vi "daub4_DWT.vi"(10 "RMS":dbl[](array[numeric])) -> (2 "Wavelet Coeff":dbl[](array[numeric]))   [LabVIEW 2014]
uses:
  <vilib>/imath/engines/lvmath2/RunTimeEngine/Managers/WorkSpace/UID Generator.vi
  <vilib>/imath/engines/lvmath2/RunTimeEngine/RunTimeType/NIMS_RunTimeType_From StrictType (excl LVString).vi
  <instcachedir>/0/NIMS_RunTimeType_From StrictType (excl LVString)_15A5391EEA9C4AACB9955AC755B83D29.lvgen/NIMS_RunTimeType_From StrictType (excl LVString)_15A5391EEA9C4AACB9955AC755B83D29_000.vi
  <vilib>/imath/engines/lvmath2/RunTimeEngine/LocalVariableDefStatement/MC_LocalVariableDefStatement_Display.vi
  <vilib>/imath/engines/lvmath2/RunTimeEngine/BuiltInFunctions/length/NIMS_length(GV).vi
  <instcachedir>/0/NIMS_length(GV)_08A3D13377FD4E4B96F5795FBF3698FA.lvgen/NIMS_length(GV)_08A3D13377FD4E4B96F5795FBF3698FA_000.vi
  <vilib>/imath/engines/lvmath2/RunTimeEngine/IndexReplace/NIMS V(R2)=V.vi
  <instcachedir>/0/NIMS V(R2)=V_680A6DA97A4E4BC09213CA62845C7083.lvgen/NIMS V(R2)=V_680A6DA97A4E4BC09213CA62845C7083_000.vi
  <vilib>/imathl/engines/lvmath/Functions/Error Handling/Create Error.vi
  <vilib>/imath/engines/lvmath2/RunTimeEngine/IndexRead/NIMS V(R2).vi
  <instcachedir>/0/NIMS V(R2)_C76619605A0E4E9F8B2FA9389712AC47.lvgen/NIMS V(R2)_C76619605A0E4E9F8B2FA9389712AC47_000.vi
  <vilib>/imath/engines/lvmath2/RunTimeEngine/ErrorHandling/NIMS_Create Error From Enums.vi
  <vilib>/imath/engines/lvmath2/RunTimeEngine/RangeToken/NIMS_Range_R2 - Float.vi
  <instcachedir>/0/NIMS_Range_R2 - Float_ED90616254C147DDA342550BD0F0CB31.lvgen/NIMS_Range_R2 - Float_ED90616254C147DDA342550BD0F0CB31_000.vi
  <vilib>/imath/engines/lvmath2/RunTimeEngine/CommandStatement/MC_CommandStatement_break.vi
  <vilib>/imath/engines/lvmath2/RunTimeEngine/VariableToken/NIMS_VariableToken_CondDefinedDefinedByReplace.vi
  <instcachedir>/0/NIMS_VariableToken_CondDefinedDefinedByReplace_D162CFFC24174562A9FEA619A91E1A56.lvgen/NIMS_VariableToken_CondDefinedDefinedByReplace_D162CFFC24174562A9FEA619A91E1A56_003.vi
  <vilib>/imath/engines/lvmath2/RunTimeSupport/NIMS_Error if Not Equal.vi
  <instcachedir>/0/NIMS_Error if Not Equal_8A0E9F659B9142D69417CC259581C4FD.lvgen/NIMS_Error if Not Equal_8A0E9F659B9142D69417CC259581C4FD_000.vi
  <vilib>/imath/engines/lvmath2/RunTimeEngine/ArithmeticOperatorToken/NIMS_ArithmeticOperator_multmx(RV,CV).vi
  <instcachedir>/0/NIMS_ArithmeticOperator_multmx(RV,CV)_944066AB0DAB474E96948A92A9572FA1.lvgen/NIMS_ArithmeticOperator_multmx(RV,CV)_944066AB0DAB474E96948A92A9572FA1_000.vi
  <vilib>/imath/engines/lvmath2/RunTimeEngine/IndexReplace/NIMS V(S)=M.vi
  <instcachedir>/0/NIMS V(S)=M_608EF2A6197B4B6A9CB600D58D177061.lvgen/NIMS V(S)=M_608EF2A6197B4B6A9CB600D58D177061_001.vi
  <vilib>/imath/engines/lvmath2/RunTimeEngine/VariableToken/NIMS_VariableToken_CondDefined.vi
  <instcachedir>/0/NIMS_VariableToken_CondDefined_EE8DD211A89249938CE6537267F5C9B3.lvgen/NIMS_VariableToken_CondDefined_EE8DD211A89249938CE6537267F5C9B3_004.vi
  <vilib>/imath/engines/lvmath2/RunTimeEngine/Managers/SymbolTable/Clear UID.vi
  <vilib>/imath/engines/lvmath2/RunTimeEngine/NodeEndStatement/NIMS_NodeEndStatement_Output.vi
  <instcachedir>/0/NIMS_NodeEndStatement_Output_53EC0D466D134D7ABD903AC30B43404B.lvgen/NIMS_NodeEndStatement_Output_53EC0D466D134D7ABD903AC30B43404B_005.vi
  <vilib>/imath/engines/lvmath2/RunTimeEngine/ErrorHandling/NIMS_Finalize Error.vi
  <vilib>/imath/engines/lvmath2/RunTimeEngine/Managers/SymbolTable/NIMS_WorkSpace.lvlib
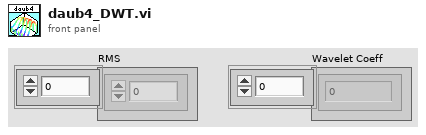
[diagram p1: front panel]
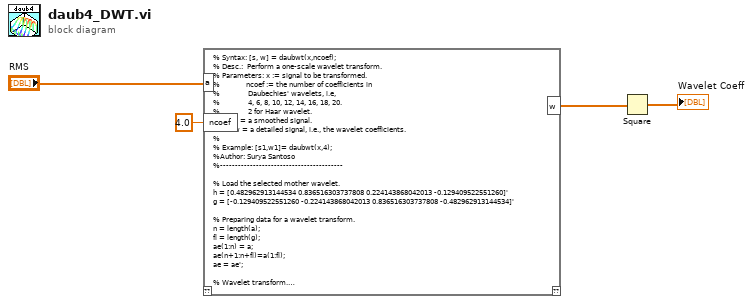
[diagram p0: block diagram]
diagram:
  n1 = mathscript code="% Syntax: [s, w] = daubwt(x,ncoef);\n% Desc.:  Perform a one-scale wavelet transform.\n% Parameters: x := signal to be transformed.\n%             ncoef := the number of coefficients in\n%\t             Daubechies' wavelets, i.e,\n%\t             4, 6, 8, 10, 12, 14, 16, 18, 20.\n%\t             2 for Haar wavelet.\n%\t      s = a smoothed signal.\n%\t      w = a detailed signal, i.e., the wavelet coefficients.\n%\n% Example: [s1,w1]= daubwt(x,4);\n%Author: Surya Santoso\n%-----------------------------------------\n\n% Load the selected mother wavelet.\nh = [0.482962913144534 0.836516303737808 0.224143868042013 -0.129409522551260]'\ng = [-0.129409522551260 -0.224143868042013 0.836516303737808 -0.482962913144534]'\n\n% Preparing data for a wavelet transform.\nn = length(a);\nfl = length(g);\nae(1:n) = a;\nae(n+1:n+fl)=a(1:fl);\nae = ae';\n\n% Wavelet transform. \ni = 1;\nfor k = 1:n/2\n    str = i;\n    stp = i+ fl - 1 ;\n    s(k) = h'*ae(str:stp);\n    w(k) = g'*ae(str:stp);\n    i = i +2;\nend\ns = s';\nw = w';"("a"="RMS", "ncoef"=4.0) -> ("w"=w3:dbl[])  [unwired: 1 in, 1 out]
  n2 = Square(x=w3) -> (x^2=→"Wavelet Coeff":dbl[])
